vi "TestSecuence.vi"(10 "String":string, 11 "Result Set":string[](array[string])) -> (0 "Time":i32, 1 "ACQType":T1 items=["Digital", "Analog"], 2 "AnalogConfig":T2, 3 "DigitalConfig":T3)   [LabVIEW 2020, in "Settings.lvlib"]
uses:
  Settings.lvlib
  Acquisition/DigitalConfig--cluster.ctl
  Acquisition/AnalogConfig--cluster.ctl
  Downloads/ProyFinSAD_PabloCesarRamosE/EnumTypeDef.ctl
  AcqType--enum.ctl
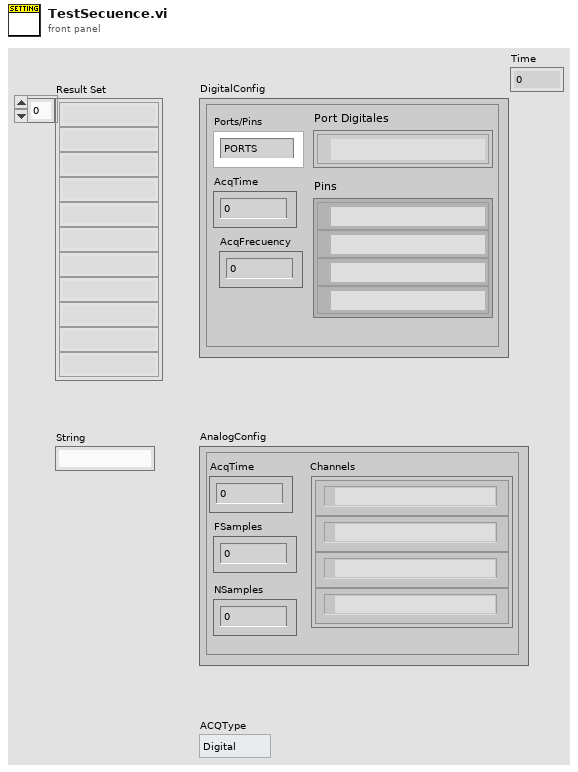
[diagram p1: front panel]
types:
  T1 = typedef "EnumTypeDef.ctl" = u16
  T2 = typedef "AnalogConfig--cluster.ctl" = cluster{"AcqTime":dbl, "FSamples":dbl, "NSamples":dbl, "Channels":tag[]}
  T3 = typedef "DigitalConfig--cluster.ctl" = cluster{"Ports/Pins":enum16{"PORTS", "PINS"}, "AcqTime":dbl, "AcqFrecuency":dbl, "Port Digitales":tag[], "Pins":tag[]}
  T4 = typedef "AcqType--enum.ctl" = enum16{"Digital", "Analog"}
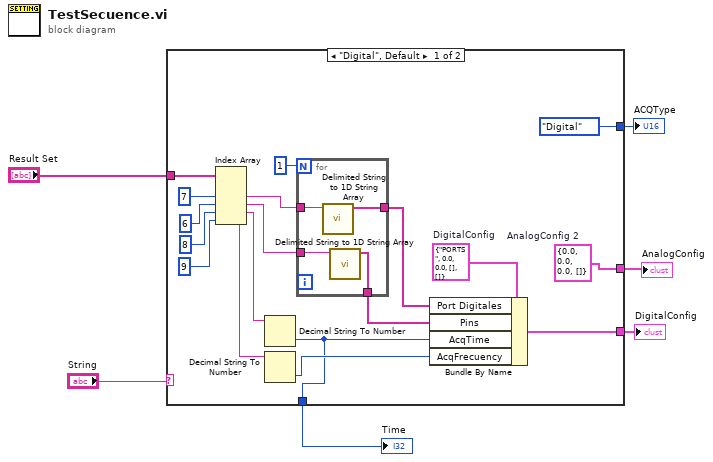
[diagram p0: block diagram]
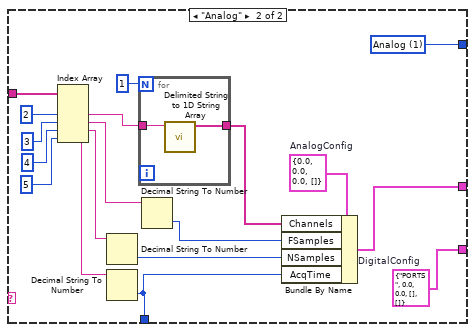
[diagram p2: hidden frame]
diagram:
  n1 = case shown="\"Digital\", Default" "String" {
    tunnel: "Result Set" -> [w24 w46]
    tunnel: [AcqType--enum."Digital" ("AcquisitionType") w36] -> w4
    tunnel: [w9 w30] -> w3
    tunnel: [w8 w31] -> w2
    tunnel: [w7 w29] -> w1
    frame "Digital", Default {
      w8 = T2 {"AcqTime"=0.0, "FSamples"=0.0, "NSamples"=0.0, "Channels"=[]}  # AnalogConfig 2
      w10 = T3 {"Ports/Pins"=enum."PORTS", "AcqTime"=0.0, "AcqFrecuency"=0.0, "Port Digitales"=[], "Pins"=[]}  # DigitalConfig
      n2 = Index Array(array=w24, index #2=7 ("index"), index #3=6 ("index"), index #4=8 ("index"), index #5=9 ("index")) -> (element #2=w17:string, element #3=w13:string, element #4=w16:string, element #5=w15:string)  [unwired: 1 in, 1 out]
      n3 = Decimal String To Number(string=w16) -> (number=w7:i32)  [unwired: 2 in, 1 out]
      n4 = Decimal String To Number(string=w15) -> (number=w14:i32)  [unwired: 2 in, 1 out]
      n5 = for {
        N: 1 -> [_]
        tunnel: w17 -> [w27]
        tunnel: [w28] -> w23
        tunnel: w13 -> [w26]
        tunnel: [w25] -> w12
        n6 = call <vilib>:"Delimited String to 1D String Array.vi"("delimited string"=w27) -> ("string array"=w28:string[])  [unwired: 10 in]
        n7 = call <vilib>:"Delimited String to 1D String Array.vi"("delimited string"=w26) -> ("string array"=w25:string[])  [unwired: 10 in]
      }
      n8 = Bundle By Name(cluster=w10, "Port Digitales"=w23, "Pins"=w12, "AcqTime"=w7, "AcqFrecuency"=w14) -> (w9:T3)
    }
    frame "Analog" {
      w30 = T3 {"Ports/Pins"=enum."PORTS", "AcqTime"=0.0, "AcqFrecuency"=0.0, "Port Digitales"=[], "Pins"=[]}  # DigitalConfig
      w32 = T2 {"AcqTime"=0.0, "FSamples"=0.0, "NSamples"=0.0, "Channels"=[]}  # AnalogConfig
      w36 = T1 1 items=["Digital", "Analog"] ("Type")
      n9 = Index Array(array=w46, index #2=2 ("index"), index #3=3 ("index"), index #4=4 ("index"), index #5=5 ("index")) -> (element #2=w39:string, element #3=w34:string, element #4=w38:string, element #5=w37:string)  [unwired: 1 in, 1 out]
      n10 = Decimal String To Number(string=w38) -> (number=w35:i32)  [unwired: 2 in, 1 out]
      n11 = Decimal String To Number(string=w37) -> (number=w29:i32)  [unwired: 2 in, 1 out]
      n12 = for {
        N: 1 -> [_]
        tunnel: w39 -> [w47]
        tunnel: [w48] -> w45
        n13 = call <vilib>:"Delimited String to 1D String Array.vi"("delimited string"=w47) -> ("string array"=w48:string[])  [unwired: 10 in]
      }
      n14 = Decimal String To Number(string=w34) -> (number=w33:i32)  [unwired: 2 in, 1 out]
      n15 = Bundle By Name(cluster=w32, "Channels"=w45, "FSamples"=w33, "NSamples"=w35, "AcqTime"=w29) -> (w31:T2)
    }
  }
  "DigitalConfig" <- w3
  "AnalogConfig" <- w2
  "ACQType" <- w4
  "Time" <- w1
